vi "Write Multiple Coils.vi"(8 "error in":errorcluster, 9 "coils":bool[](array[boolean]), 10 "starting address":u16, 11 "Master CR in":refnum<class "WebSocket Client CR.lvclass">) -> (0 "error out":errorcluster, 3 "Master CR out":refnum<class "WebSocket Client CR.lvclass">)   [LabVIEW 2021]
doc: "Writes the values of multiple coils in series, starting at address M."
uses:
  WebSocket Client CR.lvclass
  WebSocket Client CR.lvclass/WebSocket Client CR.ctl
  Modbus_v121c/Data Model/Device Data Model.lvclass
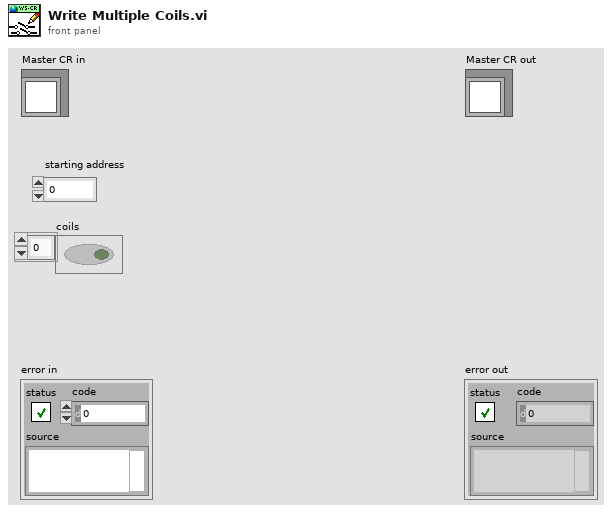
[diagram p1: front panel]
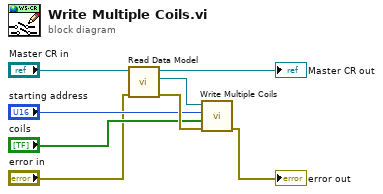
[diagram p0: block diagram]
diagram:
  n1 = call "Read Data Model.vi"("error in (no error)"="error in", "Master CR in"="Master CR in") -> ("error out"=w7:errorcluster, "Data Model"=w8:refnum<class "Device Data Model.lvclass">, "Master CR out"=→"Master CR out":refnum<class "WebSocket Client CR.lvclass">)  [unwired: 7 in]
  n2 = call-dynamic "Write Multiple Coils.vi"("error in"=w7, "coils"="coils", "starting address"="starting address", "device data model in"=w8) -> ("error out"=→"error out":errorcluster)  [unwired: 6 in, 1 out]
